vi "Dispose Report.vi"(0 "report in":refnum<class "NI_Excel.lvclass">, 5 "wait until printing completed? (T)":bool=TRUE, 9 "save changes? (F)":bool, 11 "error in (no error)":errorcluster, 12 "close report? (T)":bool=TRUE) -> (15 "error out":errorcluster)   [LabVIEW 2020, in "NI_Excel.lvclass"]
doc: "Closes the report and releases its interface, which saves memory."
uses:
  <vilib>/Utility/NIReport.llb/Excel/NI_Excel.lvclass
  <vilib>/Utility/NIReport.llb/Excel/NI_Excel.lvclass/NI_Excel.ctl
  <vilib>/addons/_office/NI_ReportGenerationToolkit.lvlib
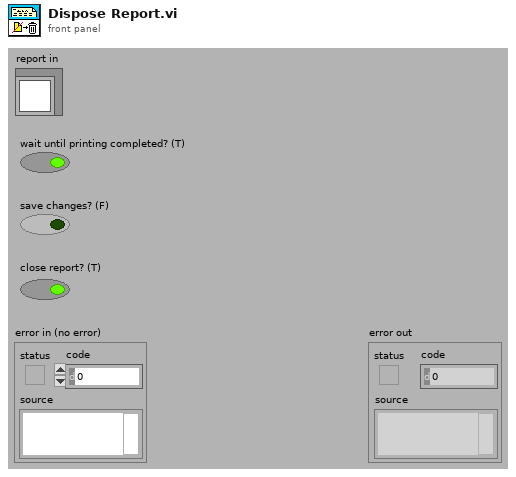
[diagram p1: front panel]
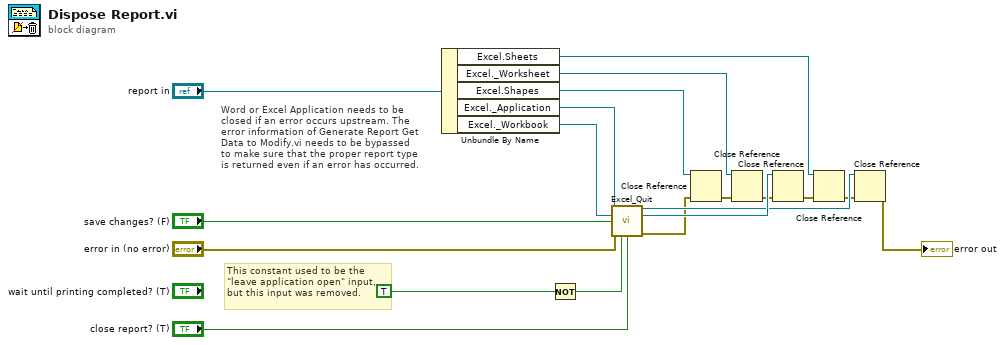
[diagram p0: block diagram]
diagram:
  # "This constant used to be the\n\"leave application open\" input,\nbut this input was removed."
  # "Word or Excel Application needs to be closed if an error occurs upstream. The error information of Generate Report Get Data to Modify.vi needs to be bypassed to make sure that the proper report type is returned even if an error has occurred."
  n1 = Unbundle By Name("report in") -> ("Excel.Sheets"=w13:refnum<k7>, "Excel._Worksheet"=w11:refnum<k7>, "Excel.Shapes"=w12:refnum<k7>, "Excel._Application"=w18:refnum<k7>, "Excel._Workbook"=w19:refnum<k7>)
  n2 = Not(x=TRUE) -> (.not. x?=w14:bool)
  n3 = call <vilib>:"Excel_Quit.vi"("Excel._Application in"=w18, "Excel._Workbook in"=w19, "save changes?"="save changes? (F)", "error in"="error in (no error)", "Close Application"=w14, "Close Report"="close report? (T)") -> ("Excel._Application out"=w16:refnum<k7>, "Excel._Workbook out"=w17:refnum<k7>, "error out"=w15:errorcluster)  [unwired: 7 out]
  n4 = Close Reference(reference=w12, error in (no error)=w15) -> (error out=w8:errorcluster)
  n5 = Close Reference(reference=w11, error in (no error)=w8) -> (error out=w9:errorcluster)
  n6 = Close Reference(reference=w17, error in (no error)=w9) -> (error out=w10:errorcluster)
  n7 = Close Reference(reference=w13, error in (no error)=w10) -> (error out=w7:errorcluster)
  n8 = Close Reference(reference=w16, error in (no error)=w7) -> (error out=→"error out":errorcluster)
